vi "New.vi"(5 "FIFO Options":T1, 7 "fifo depths (10)":u32=10, 8 "error in (no error)":errorcluster, 10 "error size (512 B)":T2=enum."512-byte", 11 "Dispatcher Interface type":refnum<class "Dispatcher Interface.lvclass">) -> (0 "error out":errorcluster, 3 "Dispatcher Interface":refnum<class "Dispatcher Interface.lvclass">)   [LabVIEW 2017, in "DSF Core.lvlib" / "Dispatcher Interface.lvclass"]
uses:
  Dispatcher Interface.lvclass
  C:/Git/DSF/Core/Classes/Interface/Interface.lvclass
  Error Queue Sizes.ctl
  Typedefs/DSF FIFO Options.ctl
  Interface.lvclass
  Framework/Framework.lvclass
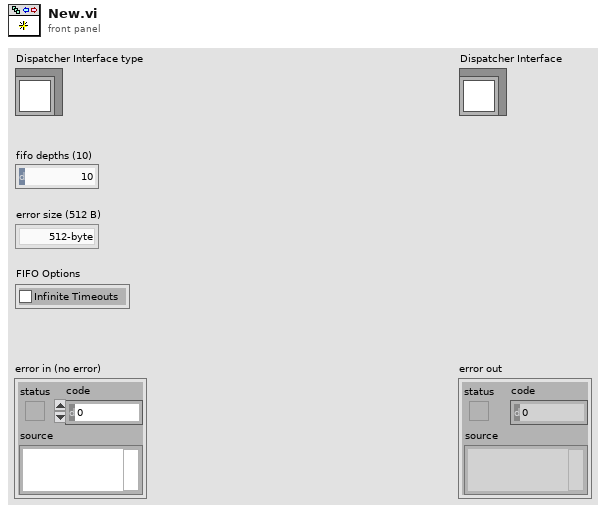
[diagram p1: front panel]
types:
  T1 = typedef "DSF Core.lvlib/Framework.lvclass/DSF FIFO Options.ctl" = cluster{"Infinite Timeouts":bool}
  T2 = typedef "DSF Core.lvlib/Interface.lvclass/Error Queue Sizes.ctl" = enum16{"256-byte", "512-byte", "1024-byte"}
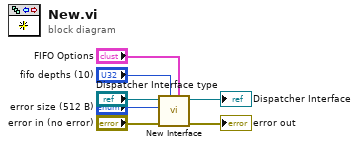
[diagram p0: block diagram]
diagram:
  n1 = call "New Interface.vi"("FIFO Options"="FIFO Options", "fifo/queue depths (10)"="fifo depths (10)", "error in (no error)"="error in (no error)", "error size (512 B)"="error size (512 B)", "Interface type"="Dispatcher Interface type") -> ("error out"=→"error out":errorcluster, "Interface"=→"Dispatcher Interface":refnum<class "Dispatcher Interface.lvclass">)  [unwired: 5 in]
